vi "LS_RANGE.vi"(6 "Heater Range":enum16{"Off", "Low", "Medium", "High"}(ring), 8 "error in (no error)":errorcluster, 9 "Heater":enum16{"A", "B"}(ring), 10 "Data Cluster In":T3 {"GUI Data Cluster"."SBR" format="%08b"}, 11 "Config Cluster In":T1={"General"={"Config.ini"=path "", "Default Logging Path"=path ""}, "Hardware"={"Measure Rate (1/s)"=0, "HP DMM VISA"="", "LS 335 VISA"="", "HP DM"={"Range"=enum."Autorange", "Autozero"=FALSE, "Display"=enum."3 1/2 Digit", "Blank LCD"=FALSE}, "LS335"={"Brightness"=enum."25%"}}, "Operation"={"Operation Mode"=enum."Logging", "Status"="", "NewLog?"=FALSE, "OvenWarn"=FALSE, "LS335"={"Heater A"={"Range"=enum."Off", "Set Point"=0.0}, "Heater B"={"Range"=enum."Off", "Set Point"=0.0}}}}) -> (0 "error out":errorcluster, 2 "Data Cluster Out":T3 {"GUI Data Cluster"."SBR" format="%08b"}, 3 "Config Cluster Out":T1={"General"={"Config.ini"=path "", "Default Logging Path"=path ""}, "Hardware"={"Measure Rate (1/s)"=0, "HP DMM VISA"="", "LS 335 VISA"="", "HP DM"={"Range"=enum."Autorange", "Autozero"=FALSE, "Display"=enum."3 1/2 Digit", "Blank LCD"=FALSE}, "LS335"={"Brightness"=enum."25%"}}, "Operation"={"Operation Mode"=enum."Idle-Off", "Status"="", "NewLog?"=FALSE, "OvenWarn"=FALSE, "LS335"={"Heater A"={"Range"=enum."Off", "Set Point"=0.0}, "Heater B"={"Range"=enum."Off", "Set Point"=0.0}}}}, 5 "return count":u32)   [LabVIEW 2021]
uses:
  Config_Cluster.ctl
  Mode_Enum.ctl
  Data_Cluster.ctl
  Measurement_Cluster.ctl
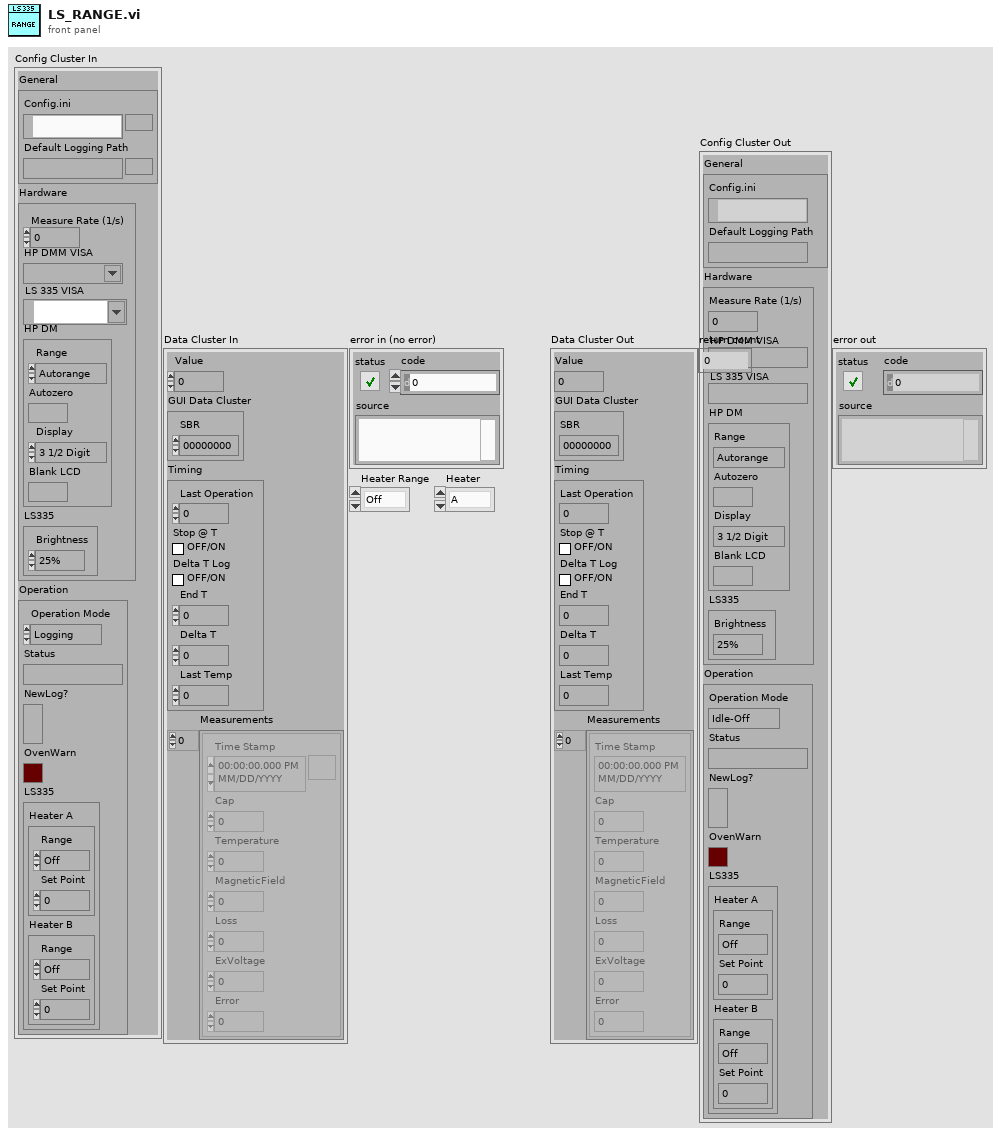
[diagram p1: front panel]
types:
  T1 = typedef "Config_Cluster.ctl" = cluster{"General":cluster{"Config.ini":path, "Default Logging Path":path}, "Hardware":cluster{"Measure Rate (1/s)":i32, "HP DMM VISA":refnum<visa-resource-name>, "LS 335 VISA":refnum<visa-resource-name>, "HP DM":cluster{"Range":enum16{"Autorange", "30mV", "300mV", "3V", "30V"}, "Autozero":bool, "Display":enum16{"3 1/2 Digit", "4 1/2 Digit", "5 1/2 Digit"}, "Blank LCD":bool}, "LS335":cluster{"Brightness":enum16{"25%", "50%", "75%", "100%"}}}, "Operation":cluster{"Operation Mode":T2, "Status":string, "NewLog?":bool, "OvenWarn":bool, "LS335":cluster{"Heater A":cluster{"Range":enum16{"Off", "Low", "Medium", "High"}, "Set Point":dbl}, "Heater B":cluster{"Range":enum16{"Off", "Low", "Medium", "High"}, "Set Point":dbl}}}}
  T2 = typedef "Mode_Enum.ctl" = enum16{"OvenNRDY", "Logging", "Idle-Off", "Idle"}
  T3 = typedef "Data_Cluster.ctl" = cluster{"Value":dbl, "GUI Data Cluster":cluster{"SBR":u16}, "Timing":cluster{"Last Operation":dbl, "Stop @ T":bool, "Delta T Log":bool, "End T":dbl, "Delta T":dbl, "Last Temp":dbl}, "Measurements":T4[]}
  T4 = typedef "Measurement_Cluster.ctl" = cluster{"Time Stamp":timestamp, "Cap":dbl, "Temperature":dbl, "MagneticField":dbl, "Loss":dbl, "ExVoltage":dbl, "Error":dbl}
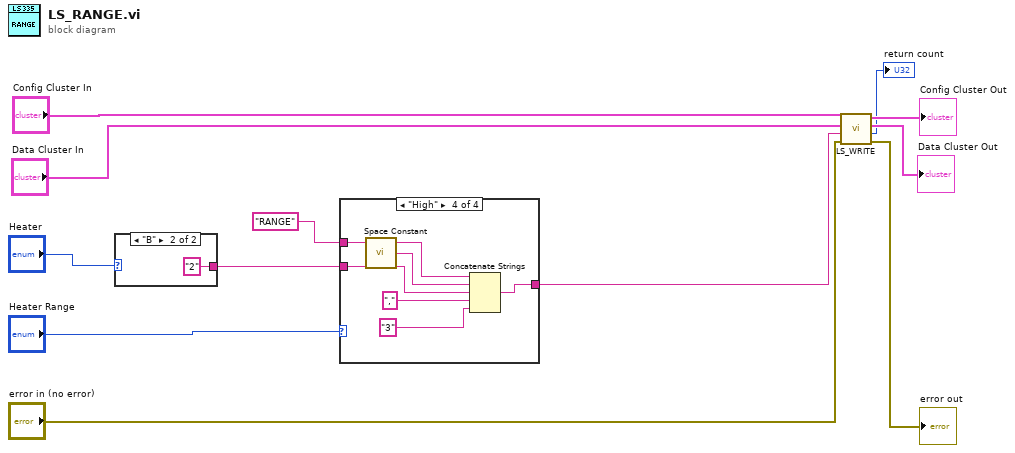
[diagram p0: block diagram]
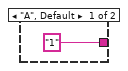
[diagram p2: hidden frame]
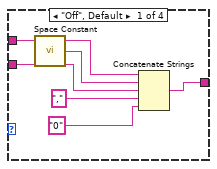
[diagram p3: hidden frame]
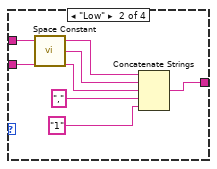
[diagram p4: hidden frame]
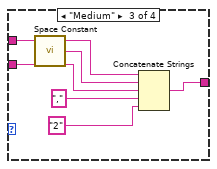
[diagram p5: hidden frame]
diagram:
  n1 = case shown="\"B\"" "Heater" {
    tunnel: ["1" "2"] -> w1
    frame "A", Default {
    }
    frame "B" {
    }
  }
  n2 = case shown="\"High\"" "Heater Range" {
    tunnel: "RANGE" -> [w20 w26 w32 w38]
    tunnel: [w18 w24 w30 w36] -> w5
    tunnel: w1 -> [w17 w23 w29 w35]
    frame "Off", Default {
      n3 = call <vilib>:"Space Constant.vi"() -> ("String"=w19:string)
      n4 = Concatenate Strings(w20, w19, w17, ",", "0") -> (w18:string)
    }
    frame "Low" {
      n5 = call <vilib>:"Space Constant.vi"() -> ("String"=w25:string)
      n6 = Concatenate Strings(w26, w25, w23, ",", "1") -> (w24:string)
    }
    frame "Medium" {
      n7 = call <vilib>:"Space Constant.vi"() -> ("String"=w31:string)
      n8 = Concatenate Strings(w32, w31, w29, ",", "2") -> (w30:string)
    }
    frame "High" {
      n9 = call <vilib>:"Space Constant.vi"() -> ("String"=w37:string)
      n10 = Concatenate Strings(w38, w37, w35, ",", "3") -> (w36:string)
    }
  }
  n11 = call "LS_WRITE.vi"("error in (no error)"="error in (no error)", "write buffer"=w5, "Data Cluster In"="Data Cluster In", "Config Cluster In"="Config Cluster In") -> ("error out"=→"error out":errorcluster, "return count"=→"return count":u32, "Data Cluster Out"=→"Data Cluster Out":T3, "Config Cluster Out"=→"Config Cluster Out":T1)  [unwired: 4 in]
